vi "Launch Logger.vi"(8 "error in (no error)":errorcluster, 11 "Worker in":refnum<class "Worker.lvclass">) -> (0 "error out":errorcluster, 3 "Worker out":refnum<class "Worker.lvclass">)   [LabVIEW 2018, in "Worker.lvclass"]
uses:
  Worker.lvclass
  C:/github/2018/LabActor/Template Module/Template Module.lvclass
  C:/Program Files/National Instruments/LabVIEW 2018/vi.lib/ActorFramework/Actor/Actor.lvclass
  Template Module/Template Module.lvclass/Template Module.ctl
  Worker.lvclass/Worker.ctl
  <vilib>/ActorFramework/Message Enqueuer/Message Enqueuer.lvclass/Message Enqueuer.ctl
  Template Module/Read Logger.vi
  Read Remote logger launched.vi
  Read Logger Enqueuer.vi
  Write Logger Enqueuer.vi
  Write Remote logger launched.vi
  <vilib>/ActorFramework/Message Enqueuer/Enqueue.vi
  Loggers/Logger/Logger.lvclass
  <vilib>/ActorFramework/Stop Msg/Stop Msg.lvclass
  C:/Program Files/National Instruments/LabVIEW 2018/vi.lib/ActorFramework/Message/Message.lvclass
  <vilib>/ActorFramework/Message Priority Queue/Priority Enqueue.vi
  <vilib>/ActorFramework/Message Enqueuer/Message Enqueuer.lvclass
  <vilib>/ActorFramework/Actor/Actor.lvclass
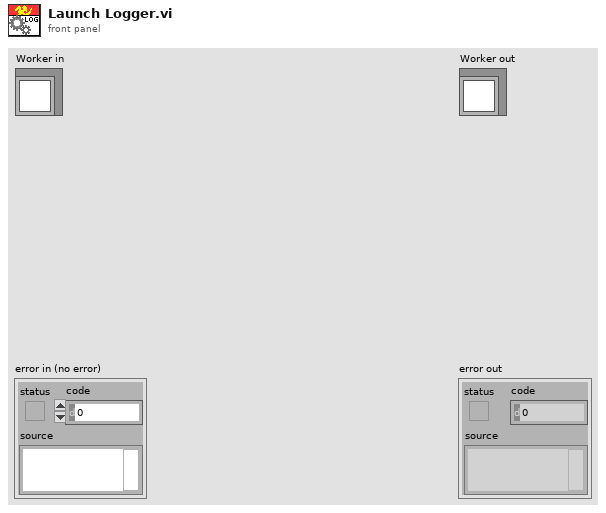
[diagram p1: front panel]
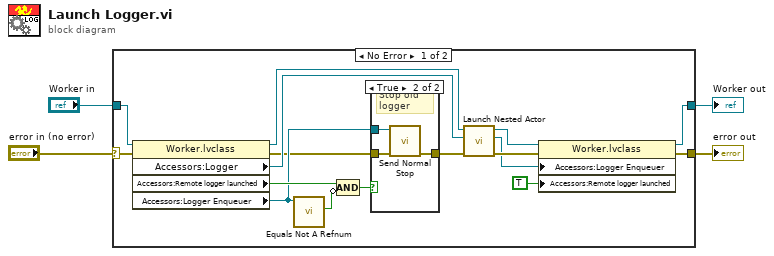
[diagram p0: block diagram]
diagram:
  n1 = case shown="No Error" "error in (no error)" {
    selector: "error in (no error)" -> [w20 w26]
    tunnel: [w15 w26] -> w3
    tunnel: [w13 w25] -> w1
    tunnel: "Worker in" -> [w19 w25]
    frame No Error {
      n2 = property class="Worker.lvclass"(reference=w19, error in=w20) -> (reference out=w17:refnum<class "Worker.lvclass">, error out=w7:errorcluster, "Accessors:Logger"=w18:refnum<class "Logger.lvclass">, "Accessors:Remote logger launched"=w10:bool, "Accessors:Logger Enqueuer"=w8:refnum<class "Message Enqueuer.lvclass">)
      n3 = call <vilib>:"Equals Not A Refnum.vi"("Message Enqueuer"=w8) -> ("Not a refnum?"=w9:bool)  [unwired: 10 in]
      n4 = Compound Arithmetic op=AND(w10, invert w9) -> (w6:bool)
      n5 = case shown="True" w6 {
        tunnel: w8 -> [_ w24]
        tunnel: w7 -> [w21 w23]
        tunnel: [w21 w22] -> w5
        frame False {
        }
        frame True {
          # "Stop old logger"
          n6 = call <vilib>:"Send Normal Stop.vi"("error in (no error)"=w23, "Message Enqueuer"=w24) -> ("error out"=w22:errorcluster)  [unwired: 9 in]
        }
      }
      n7 = call <vilib>:"Launch Nested Actor.vi"("error in (no error)"=w5, "Nested Actor"=w18, "Caller Actor in"=w17) -> ("error out"=w16:errorcluster, "Nested Actor's Enqueuer"=w12:refnum<class "Message Enqueuer.lvclass">, "Caller Actor out"=w14:refnum<class "Worker.lvclass">)  [unwired: 6 in]
      n8 = property class="Worker.lvclass"(reference=w14, error in=w16, "Accessors:Logger Enqueuer"=w12, "Accessors:Remote logger launched"=TRUE ("Remote logger launched")) -> (reference out=w13:refnum<class "Worker.lvclass">, error out=w15:errorcluster)
    }
    frame Error {
    }
  }
  "error out" <- w3
  "Worker out" <- w1
